vi "ActorNode_Create.vi"(0 "reference":refnum<class "ActorNode.lvclass">, 5 "error in (no error)":errorcluster) -> (14 "reference out":refnum<class "ActorNode.lvclass">, 19 "error out":errorcluster)   [LabVIEW 2014, in "ActorNode.lvclass"]
doc: "Creates and initializes a new ActorNode object.\n\nThis object should be destroyed using a ActorNode destructor VI or a virtual base class destructor VI.\n\n[GOOP 2.1]"
uses:
  <resource>/Framework/Providers/Open_GDS/UML/ActorNode_class/ActorNode.lvclass
  <resource>/Framework/Providers/Open_GDS/UML/MultiLineString_class/SizeType.ctl
  <resource>/Framework/Providers/Open_GDS/UML/General/Rectangle/Rectangle Rectangle2D.ctl
  <resource>/Framework/Providers/Open_GDS/UML/MultiLineString_class/JustificationType.ctl
  <resource>/Framework/Providers/Open_GDS/UML/MultiLineString_class/MultiLineString.lvclass
  <resource>/Framework/Providers/Open_GDS/UML/RectangularNode_class/RectangularNode.lvclass
panel:
  # "The input reference should only\nbe wired when this method is called\nby a sub class constructor."
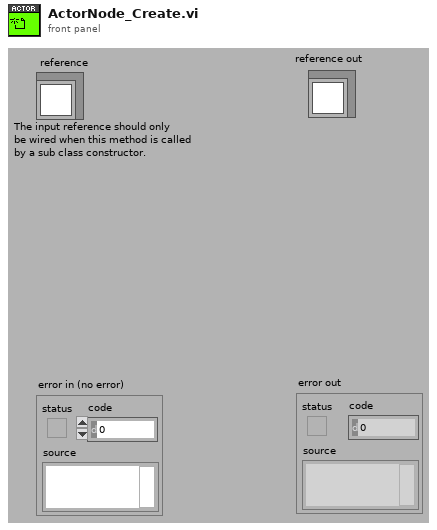
[diagram p1: front panel]
types:
  T1 = typedef "MultiLineString.lvclass/JustificationType.ctl" = enum16{"LEFT", "CENTER", "RIGHT"}
  T2 = typedef "Rectangle Rectangle2D.ctl" = cluster{"x":dbl, "y":dbl, "width":dbl, "height":dbl}
  T3 = typedef "MultiLineString.lvclass/SizeType.ctl" = enum16{"LARGE", "NORMAL", "SMALL"}
  T4 = typedef "ActorNode.lvclass/ObjectAttributes.ctl" = cluster{"name":refnum<class "MultiLineString.lvclass">, "DEFAULT_WIDTH":i32, "DEFAULT_HEIGHT":i32, "DEFAULT_GAP":i32}
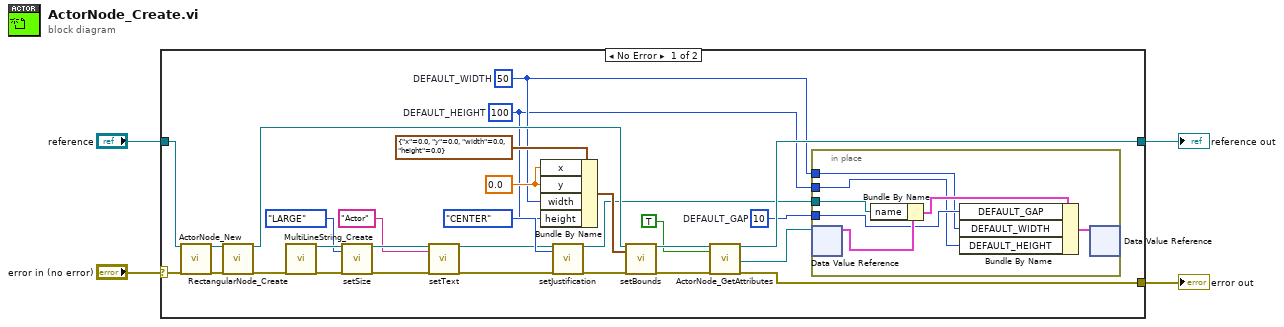
[diagram p0: block diagram]
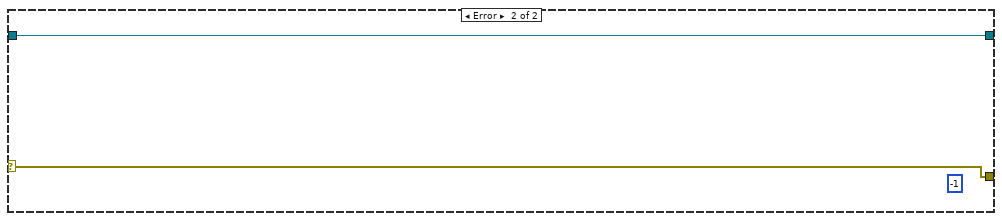
[diagram p2: hidden frame]
diagram:
  n1 = case shown="No Error" "error in (no error)" {
    selector: "error in (no error)" -> [w33 w42]
    tunnel: [w31 w41] -> w4
    tunnel: [w30 w42] -> w3
    tunnel: "reference" -> [w32 w41]
    frame No Error {
      w20 = 0.0 ("x")
      w7 = 10  # DEFAULT_GAP
      w5 = 100  # DEFAULT_HEIGHT
      w6 = 50  # DEFAULT_WIDTH
      n2 = call <resource>:"ActorNode_New.vi"("reference in"=w32, "error in (no error)"=w33) -> ("reference out"=w18:refnum<class "ActorNode.lvclass">, "error out"=w29:errorcluster)  [unwired: 2 in, 14 out]
      n3 = call <resource>:"RectangularNode_Create.vi"("reference"=w18, "error in (no error)"=w29) -> ("reference out"=w23:refnum<class "ActorNode.lvclass">, "error out"=w28:errorcluster)  [unwired: 1 in, 15 out]
      n4 = call <resource>:"MultiLineString_Create.vi"("error in (no error)"=w28) -> ("reference out"=w27:refnum<class "MultiLineString.lvclass">, "error out"=w26:errorcluster)  [unwired: 2 in, 15 out]
      n5 = call <resource>:"setSize.vi"("reference"=w27, "size"=SizeType."LARGE", "error in (no error)"=w26) -> ("reference out"=w16:refnum<class "MultiLineString.lvclass">, "error out"=w15:errorcluster)  [unwired: 15 out]
      n6 = call-dynamic "setText.vi"("reference"=w16, "text"="Actor", "error in (no error)"=w15) -> ("reference out"=w12:refnum<class "MultiLineString.lvclass">, "error out"=w13:errorcluster)  [unwired: 15 in]
      n7 = Bundle By Name(cluster=T2 {"x"=0.0, "y"=0.0, "width"=0.0, "height"=0.0} ("bounds"), "x"=w20, "y"=w20, "width"=w6, "height"=w5) -> (w22:T2)
      n8 = call <resource>:"setJustification.vi"("reference"=w12, "justification"=JustificationType."CENTER", "error in (no error)"=w13) -> ("reference out"=w8:refnum<class "MultiLineString.lvclass">, "error out"=w19:errorcluster)  [unwired: 15 out]
      n9 = call-dynamic "setBounds.vi"("reference"=w23, "bounds"=w22, "error in (no error)"=w19) -> ("reference out"=w11:refnum<class "ActorNode.lvclass">, "error out"=w17:errorcluster)  [unwired: 15 in]
      n10 = call <resource>:"ActorNode_GetAttributes.vi"("reference in"=w11, "OnlyGetDvrReference(False)"=TRUE, "error in (no error)"=w17) -> ("reference out"=w31:refnum<class "ActorNode.lvclass">, "DataRef"=w9:refnum<data-value>, "error out"=w30:errorcluster)  [unwired: 13 in, 1 out]
      n11 = in-place {
        in-place-border: w8 -> [w39]
        in-place-border: w7 -> [w37]
        in-place-border: w6 -> [w36]
        in-place-border: w5 -> [w35]
        n12 = in-place-dvr #1(w9) -> (w40:T4)  [unwired: 1 out]
        n13 = Bundle By Name(cluster=w40, "name"=w39) -> (w38:T4)
        n14 = Bundle By Name(cluster=w38, "DEFAULT_GAP"=w37, "DEFAULT_WIDTH"=w36, "DEFAULT_HEIGHT"=w35) -> (w34:T4)
        n15 = in-place-dvr #1(w34) -> ()  [unwired: 2 out]
      }
    }
    frame Error {
      (unwired) -1 ("Nr of open handles")
    }
  }
  "error out" <- w3
  "reference out" <- w4
